vi "Createpolynomial2.vi"(2 "Flyback (ms)":dbl=24.0, 3 "Acquisition time (ms)":dbl=976.0, 4 "Save calibration":bool, 11 "P(x)":dbl[](array[numeric])=[-2.759061878613649, 0.19366471754794023, 3.230876995543825, -0.29433534392220473, 116.96354405008198, -108.15732631503944, 0.6433055492502915] step=1e-10 format="%#.33f") -> (0 "Generate two signals":dbl[](graph))   [LabVIEW 2020]
panel:
  out "Descending voice coil motion":dbl[](graph)=[0.9300488575312627, 0.9294735374146255, 0.9288775134189357, 0.9282608286657484, 0.9276235277713978, 0.9269656568437696, 0.9262872634789617, 0.9255883967578462, 0.9248691072425148, 0.9241294469726217, 0.9233694694616184, 0.9225892296928823, 0.9217887841157384, 0.9209681906413758, 0.9201275086386571, 0.9192667989298255, 0.918386123786098, 0.9174855469231689, 0.9165651334965945, 0.9156249500970803, 0.9146650647456638, 0.9136855468887923, 0.9126864673933, 0.9116678985412792, 0.910629914024854, 0.9095725889408408, 0.9084959997853259, 0.9074002244481245, 0.9062853422071466, 0.9051514337226619, 0.9039985810314638, 0.9028268675409341, 0.901636378023009, 0.9004271986080473, 0.8991994167785919, 0.8979531213630516, 0.896688402529267, 0.8954053517779887, 0.8941040619362581, 0.8927846271506903, 0.8914471428806636, 0.8900917058914126, 0.8887184142470279, 0.8873273673033634, 0.8859186657008382, 0.8844924113571704, 0.8830487074599931, 0.881587658459392, 0.8801093700603484, 0.8786139492150912, 0.8771015041153596, 0.8755721441845751, 0.8740259800699278, 0.8724631236343607, 0.8708836879484922, 0.8692877872824248, 0.8676755370974814, 0.8660470540378503, 0.8644024559221477, 0.862741861734893, 0.8610653916178999, 0.859373166861585, 0.8576653098961959, 0.8559419442829407, 0.8542031947050666, 0.8524491869588278, 0.850680047944387, 0.8488959056566343, 0.8470968891759267, 0.84528312865875, 0.8434547553283014, 0.8416119014649993, 0.8397547003969003, 0.8378832864900717, 0.8359977951388582, 0.8340983627560887, 0.8321851267632081, 0.8302582255803338, 0.8283177986162422, 0.8263639862582821, 0.8243969298622214, 0.8224167717420067, 0.8204236551594872, 0.8184177243140368, 0.8163991243321241, 0.8143680012568135, 0.8123245020371985, 0.8102687745177708, 0.8082009674277231, 0.8061212303701896, 0.8040297138114253, 0.8019265690699063, 0.799811948305403, 0.7976860045079575, 0.7955488914868183, 0.793400763859313, 0.7912417770396611, 0.7890720872277308, 0.7868918513977375, 0.7847012272868912, 0.7825003733839689, 0.7802894489178711, 0.7780686138460866, 0.7758380288431233, 0.773597855288884, 0.7713482552569908, 0.7690893915030588, 0.7668214274529215, 0.7645445271908068, 0.7622588554474695, 0.7599645775882585, 0.757661859601175, 0.7553508680848489, 0.7530317702364886, 0.7507047338397855, 0.7483699272527744, 0.7460275193956533, 0.7436776797385617, 0.7413205782893246, 0.7389563855811361, 0.7365852726602453, 0.7342074110735658, 0.7318229728562683, 0.7294321305193341, 0.7270350570370742, 0.7246319258346148, 0.7222229107753502, 0.719808186148368, 0.7173879266558236, 0.7149623074003246, 0.7125315038722466, 0.7100956919370404, 0.7076550478225084, 0.705209748106055, 0.7027599697019112, 0.7003058898483354, 0.69784768609479, 0.6953855362891002, 0.6929196185645707, 0.6904501113271229, 0.6879771932423698, 0.6855010432226956, 0.68302184041431, 0.6805397641842887, 0.6780549941075952, 0.6755677099540893, 0.6730780916755253, 0.6705863193925159, 0.6680925733815255, 0.6655970340618111, 0.6630998819823735, 0.6606012978088939, 0.6581014623106642, 0.6556005563475078, 0.6530987608566948, 0.6505962568398517, 0.6480932253498697, 0.6455898474777897, 0.6430863043397255, 0.6405827770637433, 0.638079446776762, 0.6355764945914482, 0.6330741015931136, 0.6305724488266133, 0.628071717283248, 0.6255720878876727, 0.6230737414847913, 0.6205768588266973, 0.6180816205595799, 0.6155882072106591, 0.613096799175124, 0.6106075767030823, 0.6081207198865187, 0.6056364086462662, 0.6031548227189925, 0.6006761416441802, 0.598200544751162, 0.5957282111461301, 0.5932593196991818, 0.5907940490313791, 0.5883325775018252, 0.5858750831947606, 0.583421743906679, 0.580972737133464, 0.5785282400575512, 0.5760884295350938, 0.5736534820831907, 0.5712235738671003, 0.5687988806874988, 0.5663795779677612, 0.5639658407412699, 0.5615578436387512, 0.5591557608756408, 0.556759766239484, 0.5543700330773456, 0.5519867342832935, 0.549610042285873, 0.5472401290356368, 0.5448771659927036, 0.5425213241143543, 0.5401727738426623, 0.5378316850921632, 0.5354982272375611, 0.5331725691014789, 0.530854878942228, 0.5285453244416594, 0.5262440726930153, 0.5239512901888451, 0.5216671428089594, 0.5193917958084288, 0.5171254138056278, 0.5148681607703256, 0.5126202000118257, 0.5103816941671366, 0.5081528051892275, 0.5059336943352959, 0.5037245221551051, 0.5015254484793681, 0.4993366324081845, 0.4971582322995297, 0.4949904057577976, 0.4928333096224024, 0.49068709995641624, 0.48855193203530045, 0.48642796033565705, 0.48431533852405595, 0.48221421944591764, 0.4801247551144549, 0.4780470966996748, 0.4759813945174418, 0.47392779801860274, 0.47188645577817734, 0.46985751548459564, 0.4678411239290333, 0.4658374269947779, 0.46384656964667764, 0.4618686959206536, 0.45990394891327874, 0.4579524707714251, 0.45601440268197985]
  out "Add flyback to rising of voice coil":dbl[](graph)
  out "size(s) 2":i32=10000
  out "InitialPosition":dbl=0.4718151169301761
  out "EndPosition":dbl=0.9575466974300837
  out "Exponential decay ascending voice coil motion":dbl[](graph)
  # "-2.757339075566779 * np.exp(-.19284360288085645 * x) + 3.2261411630577483,\nlambda x: -0.29308107 * np.sin(116.85160518 * x - 108.06281071) + 0.64308107])"
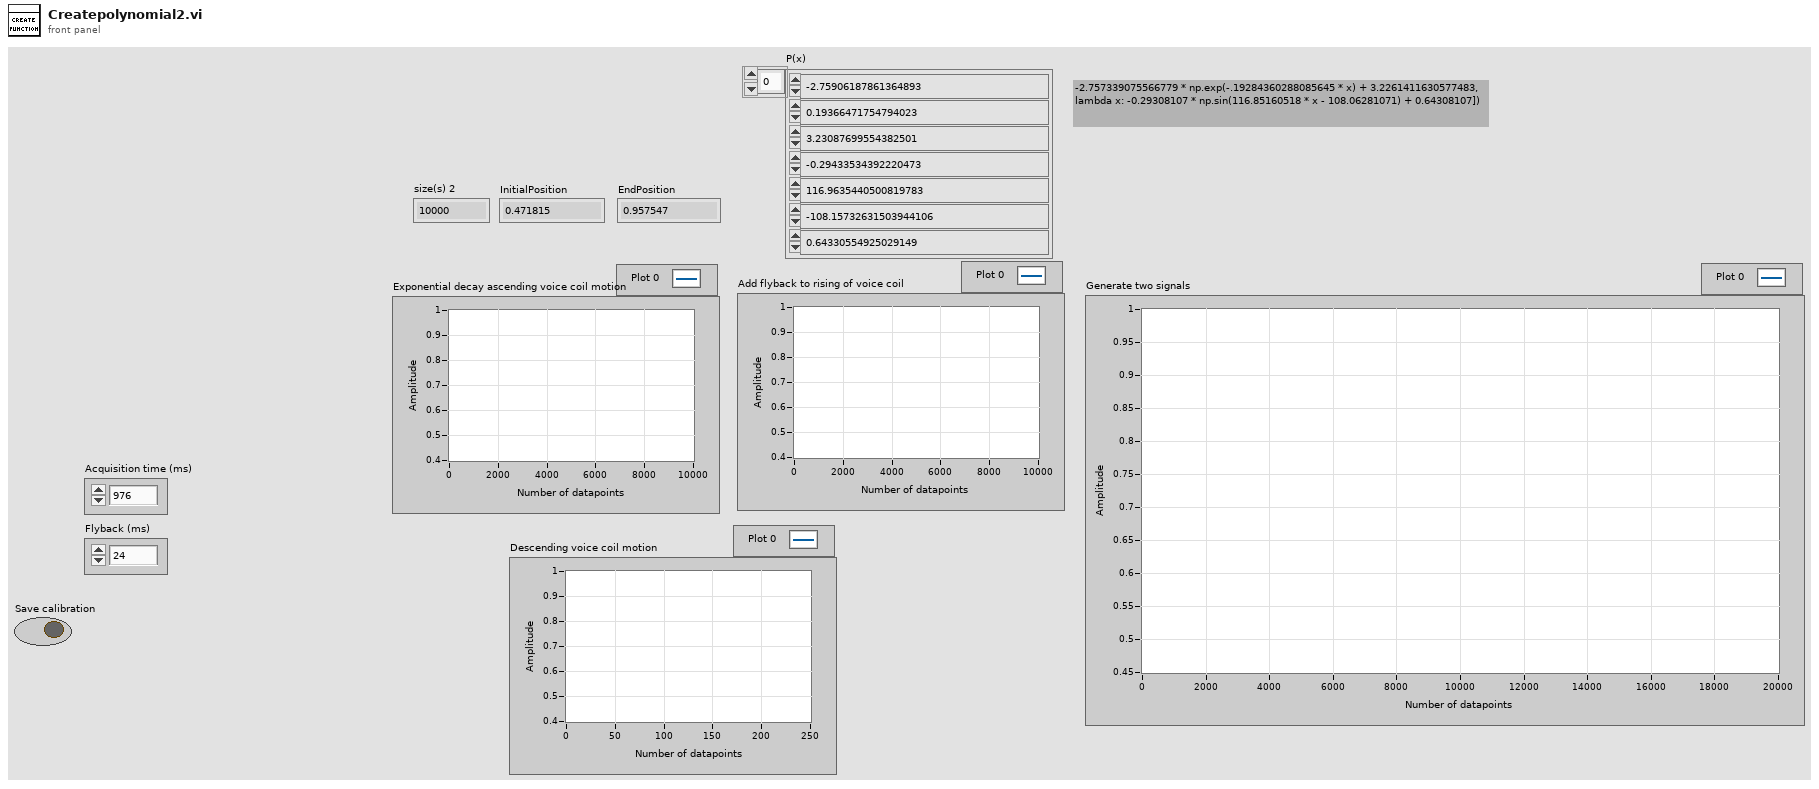
[diagram p1: front panel]
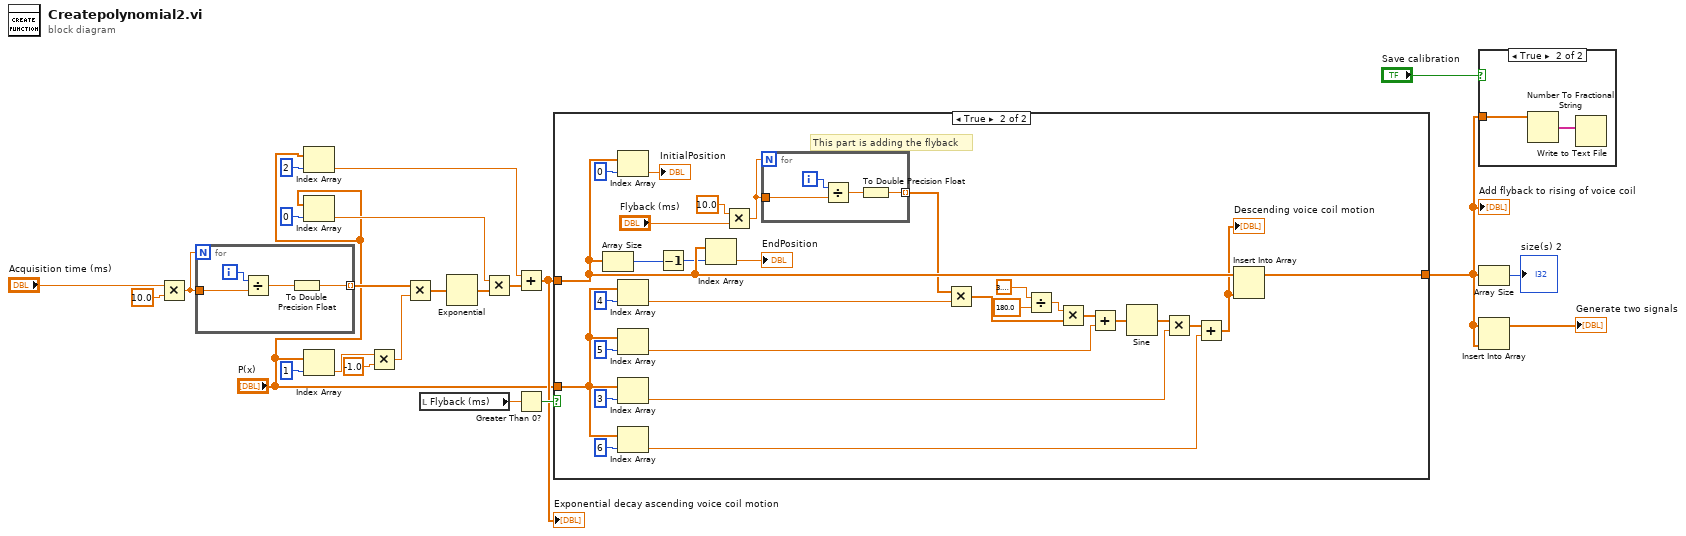
[diagram p0: block diagram]
diagram:
  n1 = Multiply(x="Acquisition time (ms)", y=10.0) -> (x*y=w16:dbl)
  n2 = for {
    N: w16 -> [_]
    tunnel: [w27] -> w12 mode=indexing
    tunnel: w16 -> [w24]
    i -> [w26]
    n3 = Divide(x=w26, y=w24) -> (x/y=w25:dbl)
    n4 = To Double Precision Float(number=w25) -> (double precision float=w27:dbl)
  }
  n5 = Index Array(array="P(x)", index=2) -> (element=w2:dbl)
  n6 = Index Array(array="P(x)", index=0) -> (element=w6:dbl)
  n7 = Index Array(array="P(x)", index=1) -> (element=w4:dbl)
  n8 = Multiply(x=w4, y=-1.0) -> (x*y=w10:dbl)
  n9 = Multiply(x=w12, y=w10) -> (x*y=w13:dbl[])
  n10 = local read "Flyback (ms)"() -> (w23:dbl)
  n11 = Exponential(1:w13) -> (0:w14:dbl[])
  n12 = Multiply(x=w6, y=w14) -> (x*y=w9:dbl[])
  n13 = Add(x=w2, y=w9) -> (x+y=w8:dbl[])
  "Exponential decay ascending voice coil motion" <- w8
  n14 = Greater Than 0?(x=w23) -> (x > 0?=w22:bool)
  n15 = case shown="True" w22 {
    tunnel: w8 -> [w28 w57]
    tunnel: [w28 w52] -> w15
    tunnel: "P(x)" -> [_ w29]
    frame False {
    }
    frame True {
      # "This part is adding the flyback"
      n16 = Array Size(array=w57) -> (size(s)=w55:i32)
      n17 = Index Array(array=w57, index=0) -> (element=→"InitialPosition":dbl)
      n18 = Index Array(array=w29, index=4) -> (element=w35:dbl)
      n19 = Index Array(array=w29, index=5) -> (element=w33:dbl)
      n20 = Index Array(array=w29, index=3) -> (element=w32:dbl)
      n21 = Index Array(array=w29, index=6) -> (element=w30:dbl)
      n22 = Decrement(x=w55) -> (x-1=w54:i32)
      n23 = Index Array(array=w57, index=w54) -> (element=→"EndPosition":dbl)
      n24 = Multiply(x=10.0, y="Flyback (ms)") -> (x*y=w46:dbl)
      n25 = for {
        N: w46 -> [_]
        tunnel: [w61] -> w43 mode=indexing
        tunnel: w46 -> [w58]
        i -> [w59]
        n26 = Divide(x=w59, y=w58) -> (x/y=w60:dbl)
        n27 = To Double Precision Float(number=w60) -> (double precision float=w61:dbl)
      }
      n28 = Multiply(x=w43, y=w35) -> (x*y=w42:dbl[])
      n29 = Divide(x=3.141592653589793, y=180.0) -> (x/y=w41:dbl)
      n30 = Multiply(x=w41, y=w42) -> (x*y=w40:dbl[])
      n31 = Add(x=w40, y=w33) -> (x+y=w39:dbl[])
      n32 = Sine(x=w39) -> (sin(x)=w38:dbl[])
      n33 = Multiply(x=w38, y=w32) -> (x*y=w48:dbl[])
      n34 = Add(x=w48, y=w30) -> (x+y=w47:dbl[])
      "Descending voice coil motion" <- w47
      n35 = Insert Into Array "Insert Into Array"(array=w57, new element=w47) -> (w52:dbl[])  [unwired: 1 in]
    }
  }
  "Add flyback to rising of voice coil" <- w15
  n36 = case shown="True" "Save calibration" {
    tunnel: w15 -> [_ w63]
    frame False {
    }
    frame True {
      n37 = Number To Fractional String(number=w63) -> (F-format string=w62:string[])  [unwired: 3 in]
      n38 = Write to Text File(text=w62) -> ()  [unwired: 3 in, 3 out]
    }
  }
  n39 = Array Size(array=w15) -> (size(s)=→"size(s) 2":i32)
  n40 = Insert Into Array "Insert Into Array"(array=w15, new element=w15) -> (→"Generate two signals":dbl[])  [unwired: 1 in]
